vi "mod_Estimate AM-SSB frequency and phase offset.vi"(0 "extracted pilot tone signal":cdb[](array[numeric]), 5 "pilot tone":dbl, 11 "error in (no error)":errorcluster, 13 "reset? (T)":bool=TRUE) -> (4 "frequency offset":dbl, 6 "phase offset (radians)":dbl, 15 "error out":errorcluster)   [LabVIEW 2020, in "niAMT.lvlib"]
uses:
  <vilib>/addons/Modulation/niAMT.lvlib
  <vilib>/Analysis/1siggen.llb/Ramp Pattern by Samples.vi
  <vilib>/Analysis/NI_AALPro.lvlib
  <vilib>/Analysis/NI_AALBase.lvlib
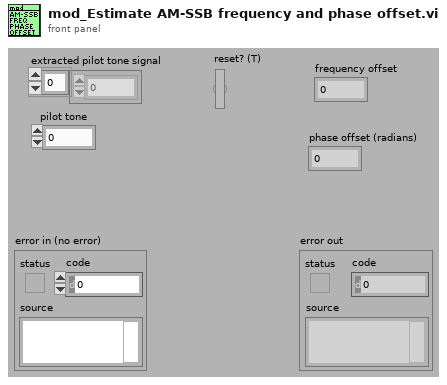
[diagram p1: front panel]
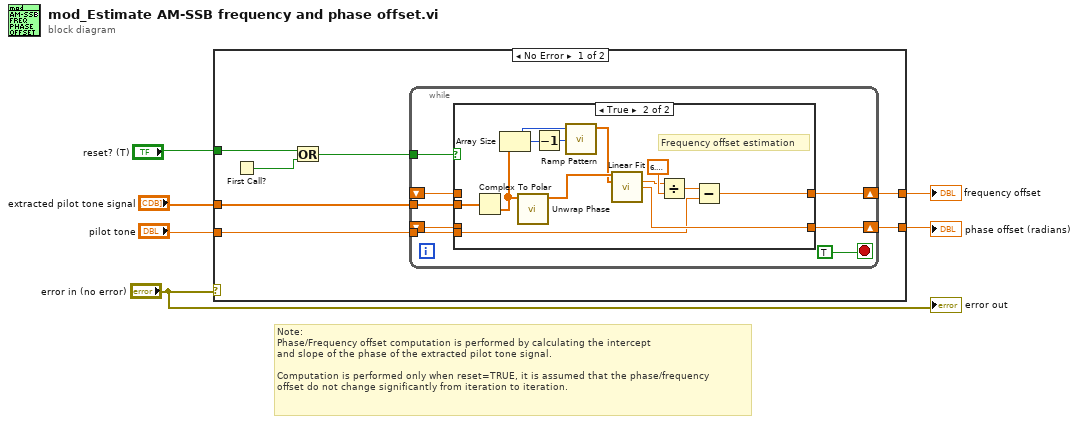
[diagram p0: block diagram]
diagram:
  # "Note:\nPhase/Frequency offset computation is performed by calculating the intercept\nand slope of the phase of the extracted pilot tone signal.\n\nComputation is performed only when reset=TRUE, it is assumed that the phase/frequency\noffset do not change significantly from iteration to iteration."
  n1 = case shown="No Error" "error in (no error)" {
    tunnel: "extracted pilot tone signal" -> [w12 _]
    tunnel: "pilot tone" -> [w11 _]
    tunnel: "reset? (T)" -> [w10 _]
    tunnel: [w8 _] -> w2
    tunnel: [w7 _] -> w1
    frame No Error {
      n2 = First Call?() -> (First Call?: T/F=w13:bool)
      n3 = Or(x=w10, y=w13) -> (x .or. y?=w9:bool)
      n4 = while {
        tunnel: w9 -> [w21]
        tunnel: w12 -> [w20]
        shift-right: [w18] -> w7
        shift-left: _ -> [w17]
        shift-right: [w16] -> w8
        shift-left: _ -> [w15]
        tunnel: w11 -> [w14]
        stop <- TRUE stop-if-true
        n5 = case shown="True" w21 {
          tunnel: w20 -> [_ w35]
          tunnel: [w23 w28] -> w18
          tunnel: w17 -> [w23 _]
          tunnel: [w22 w30] -> w16
          tunnel: w15 -> [w22 _]
          tunnel: w14 -> [_ w29]
          frame False {
          }
          frame True {
            # "Frequency offset estimation"
            n6 = Complex To Polar(r * e^(i*theta)=w35) -> (theta=w27:dbl[])  [unwired: 1 out]
            n7 = Array Size(array=w27) -> (size(s)=w26:i32)
            n8 = call <vilib>:"Unwrap Phase.vi"("Phase"=w27) -> ("Unwrapped Phase"=w31:dbl[])  [unwired: 1 in, 9 out]
            n9 = Decrement(x=w26) -> (x-1=w25:i32)
            n10 = call-poly <vilib>:"Ramp Pattern.vi"("end"=w25, "samples"=w26) -> ("Ramp Pattern"=w24:dbl[])  [unwired: 8 in, 1 out]
            n11 = call <vilib>:"Linear Fit.vi"("Y"=w31, "X"=w24) -> ("slope"=w33:dbl, "intercept"=w30:dbl)  [unwired: 4 in, 8 out]
            n12 = Divide(x=w33, y=6.283185307179586) -> (x/y=w32:dbl)
            n13 = Subtract(x=w32, y=w29) -> (x-y=w28:dbl)
          }
        }
      }
    }
    frame Error {
    }
  }
  "phase offset (radians)" <- w2
  "frequency offset" <- w1
  "error out" <- "error in (no error)"
